vi "runtest check sequence.vi"(6 "username (\"\")":string, 7 "POST (empty)":T1, 8 "error in (no error)":errorcluster, 10 "Sequence ID (\"\")":string, 11 "Connection Refnum":T2) -> (0 "error out":errorcluster, 1 "Sequence Owner?":bool, 3 "Connection Refnum":T2, 5 "POST out":T1)   [LabVIEW 2011]
uses:
  Summitek EXT/ODBC/SQL Controls/Connection Refnum.ctl
  ITK EXT/utils/keyedarr.llb/Keyed Array.ctl
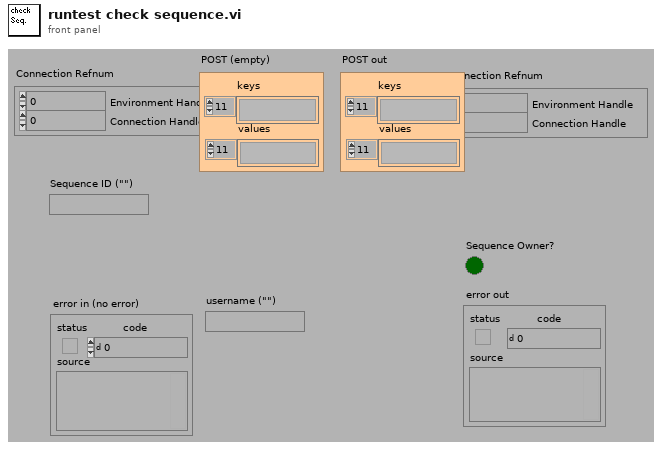
[diagram p1: front panel]
types:
  T1 = typedef "Keyed Array.ctl" = cluster{"keys":string[], "values":string[]}
  T2 = typedef "Connection Refnum.ctl" = cluster{"Environment Handle":i32, "Connection Handle":i32}
  T3 = typedef "Sequence Record.ctl" = cluster{"ixSequence":i32, "sxSequenceId":string, "sDescription":string, "sCreator":string, "tCreationDate":timestamp, "sModifier":string, "tModifiedDate":timestamp, "fApproved":bool, "fSpartanSetsSN":bool, "fOverwriteData":bool, "fStopOnFail":bool, "fDisableQuickMode":bool, "fPartialExecution":bool, "fAutoNextItem":bool, "fDoNotPrintOnFail":bool}
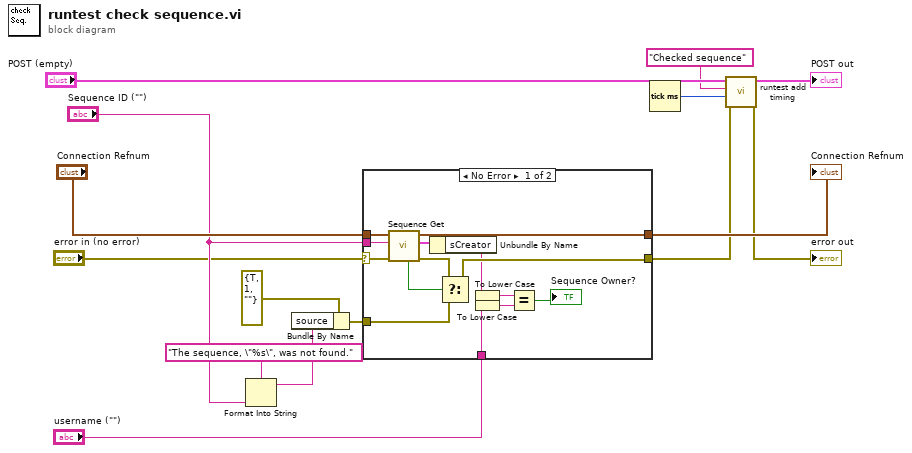
[diagram p0: block diagram]
diagram:
  n1 = Format Into String(format string="The sequence, \"%s\", was not found.", "Sequence ID (\"\")") -> (resulting string=w10:string)  [unwired: 2 in, 1 out]
  n2 = Bundle By Name(cluster=errorcluster {"status"=TRUE, "code"=1, "source"=""} ("f"), "source"=w10) -> (w12:errorcluster)
  n3 = case shown="No Error" "error in (no error)" {
    selector: "error in (no error)" -> [w22 w31]
    tunnel: "Connection Refnum" -> [w29 w30]
    tunnel: [w28 w30] -> w14
    tunnel: [w25 w31] -> w2
    tunnel: w12 -> [w24 _]
    tunnel: "Sequence ID (\"\")" -> [w23 _]
    tunnel: "username (\"\")" -> [w17 _]
    frame No Error {
      n4 = call "Sequence Get.vi"("error in (no error)"=w22, "sxSequenceId (\"\")"=w23, "Connection Refnum"=w29) -> ("error out"=w26:errorcluster, "Sequence Record"=w19:T3, "Connection Refnum"=w28:T2, "Data Present"=w27:bool)  [unwired: 5 out]
      n5 = Unbundle By Name(w19) -> ("sCreator"=w18:string)
      n6 = Select(t=w26, s=w27, f=w24) -> (s? t:f=w25:errorcluster)
      n7 = To Lower Case(string=w18) -> (all lower case string=w20:string)
      n8 = To Lower Case(string=w17) -> (all lower case string=w21:string)
      n9 = Equal?(x=w20, y=w21) -> (x = y?=→"Sequence Owner?":bool)
    }
    frame Error {
    }
  }
  "Connection Refnum" <- w14
  n10 = Tick Count (ms)() -> (millisecond timer value=w3:u32)
  n11 = call "runtest add timing.vi"("error in (no error)"=w2, "Start Tick, ms (0)"=w3, "Function (\"\")"="Checked sequence", "POST (empty)"="POST (empty)") -> ("error out"=→"error out":errorcluster, "POST out"=→"POST out":T1)  [unwired: 6 out]
